vi "Write Log file ref.vi"(10 "Log file ref":refnum<file>, 11 "BuildManager in":refnum<class "BuildManager.lvclass">) -> (3 "BuildManager out":refnum<class "BuildManager.lvclass">)   [LabVIEW 2019, in "SolutionBuilder.lvlib" / "BuildManager.lvclass"]
uses:
  BuildManager.lvclass
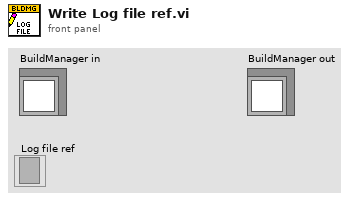
[diagram p1: front panel]
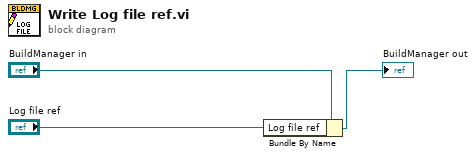
[diagram p0: block diagram]
diagram:
  n1 = Bundle By Name(cluster="BuildManager in", "Log file ref"="Log file ref") -> (→"BuildManager out":refnum<class "BuildManager.lvclass">)
